vi "LVClient_up.vi"() -> ()   [LabVIEW 2018]
uses:
  <vilib>/picture/picture.llb/imagedata.ctl
panel:
  out "?":picture
  out "image data":T1
  in  "Stop Server":bool
  in  "Stop Client":bool
  in  "Init Button":bool
  in  "Play Button":bool
  out "Python server reply (9 bytes)":string
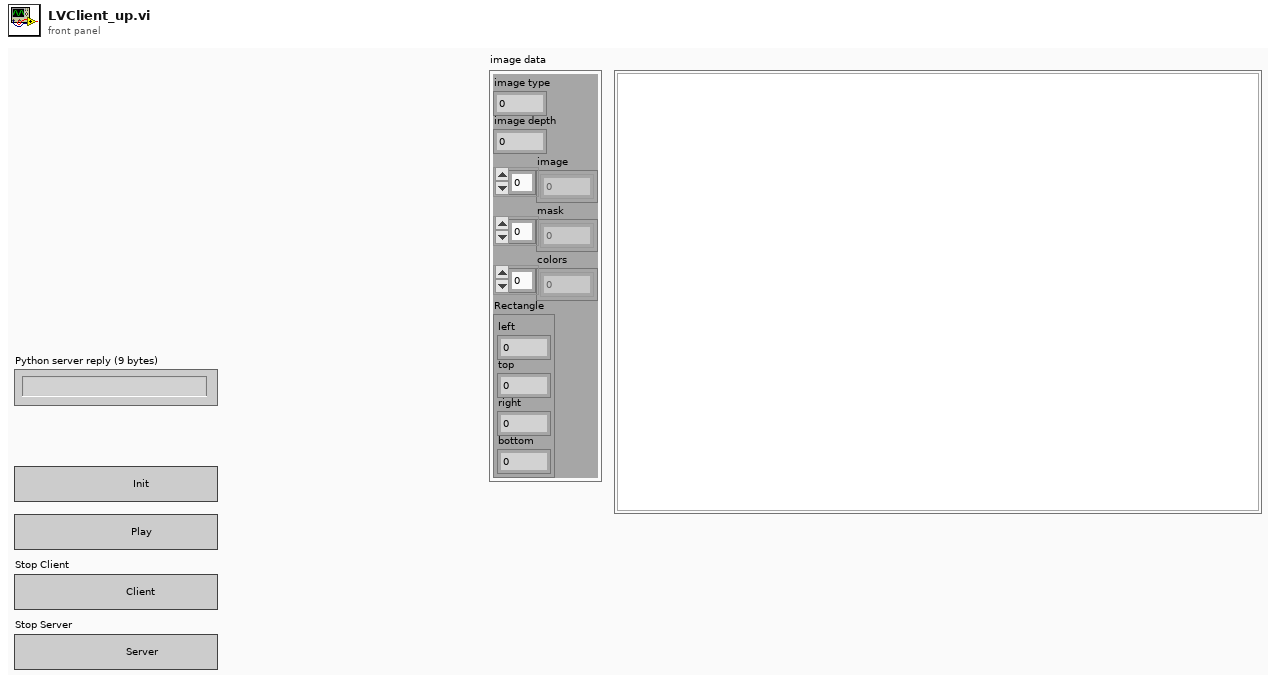
[diagram p1: front panel]
types:
  T1 = typedef "imagedata.ctl" = cluster{"image type":i32, "image depth":i32, "image":u8[], "mask":u8[], "colors":u32[], "Rectangle":cluster{"left":i16, "top":i16, "right":i16, "bottom":i16}}
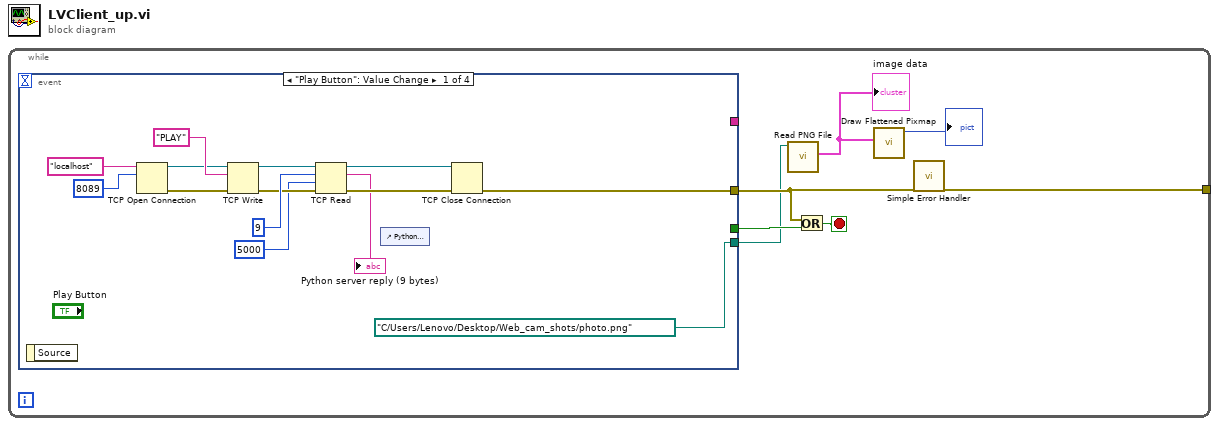
[diagram p0: block diagram]
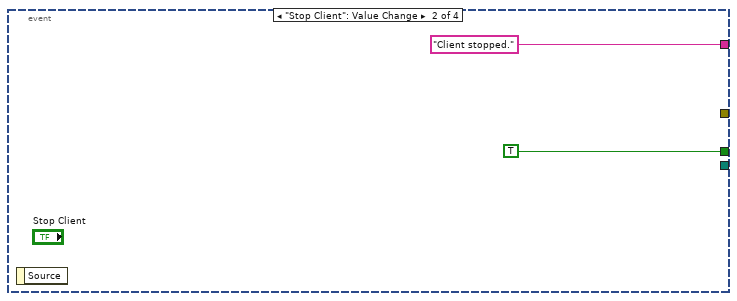
[diagram p2: hidden frame]
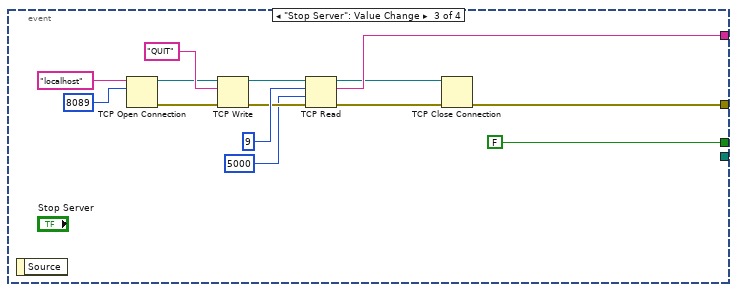
[diagram p3: hidden frame]
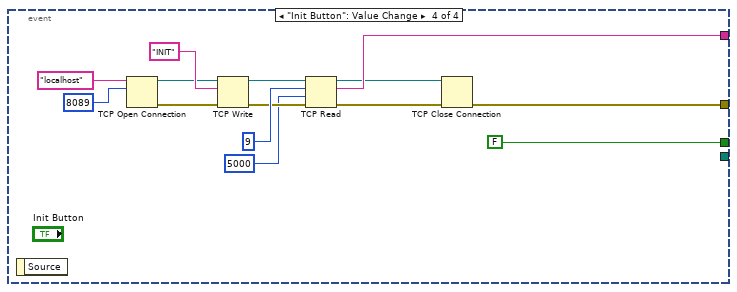
[diagram p4: hidden frame]
diagram:
  n1 = while {
    tunnel: [w7] -> w1
    stop <- w6 stop-if-true
    n2 = event shown="[0] \"Play Button\": Value Change" {
      selector: _ -> [_ _ _ _]
      dyn-events: _ -> [_ _ _ _]
      timeout: _ -> [_ _ _ _]
      tunnel: [w10 _ w25 w39] -> w7
      tunnel: [_ "Client stopped." ("data out") w32 w46] -> _
      tunnel: [_ TRUE FALSE FALSE] -> w5
      tunnel: [path "C:/Users/Lenovo/Desktop/Web_cam_shots/photo.png" _ _ _] -> w2
      event "Play Button": Value Change {
        n3 = event-data() -> ()  [unwired: 1 in, 1 out]
        n4 = TCP Open Connection(address="localhost", remote port or service name=u16 8089) -> (connection ID=w14:refnum<k5>, error out=w13:errorcluster)  [unwired: 3 in]
        n5 = TCP Write(connection ID=w14, data in="PLAY", error in (no error)=w13) -> (connection ID out=w19:refnum<k5>, error out=w18:errorcluster)  [unwired: 1 in, 1 out]
        n6 = TCP Read(connection ID=w19, bytes to read=9, error in (no error)=w18, 9:5000 ("timeout ms (25000)")) -> (connection ID out=w12:refnum<k5>, data out=→"Python server reply (9 bytes)":string, error out=w11:errorcluster)  [unwired: 1 in]
        n7 = control-ref of="Python server reply (9 bytes)"() -> ()  [unwired: 1 out]
        n8 = TCP Close Connection(connection ID=w12, error in (no error)=w11) -> (error out=w10:errorcluster)  [unwired: 1 in, 1 out]
      }
      event "Stop Client": Value Change {
        n9 = event-data() -> ()  [unwired: 1 in, 1 out]
      }
      event "Stop Server": Value Change {
        n10 = event-data() -> ()  [unwired: 1 in, 1 out]
        n11 = TCP Open Connection(address="localhost", remote port or service name=u16 8089) -> (connection ID=w29:refnum<k5>, error out=w28:errorcluster)  [unwired: 3 in]
        n12 = TCP Write(connection ID=w29, data in="QUIT", error in (no error)=w28) -> (connection ID out=w35:refnum<k5>, error out=w34:errorcluster)  [unwired: 1 in, 1 out]
        n13 = TCP Read(connection ID=w35, bytes to read=9, error in (no error)=w34, 9:5000 ("timeout ms (25000)")) -> (connection ID out=w27:refnum<k5>, data out=w32:string, error out=w26:errorcluster)  [unwired: 1 in]
        n14 = TCP Close Connection(connection ID=w27, error in (no error)=w26) -> (error out=w25:errorcluster)  [unwired: 1 in, 1 out]
      }
      event "Init Button": Value Change {
        n15 = event-data() -> ()  [unwired: 1 in, 1 out]
        n16 = TCP Open Connection(address="localhost", remote port or service name=u16 8089) -> (connection ID=w43:refnum<k5>, error out=w42:errorcluster)  [unwired: 3 in]
        n17 = TCP Write(connection ID=w43, data in="INIT", error in (no error)=w42) -> (connection ID out=w49:refnum<k5>, error out=w48:errorcluster)  [unwired: 1 in, 1 out]
        n18 = TCP Read(connection ID=w49, bytes to read=9, error in (no error)=w48, 9:5000 ("timeout ms (25000)")) -> (connection ID out=w41:refnum<k5>, data out=w46:string, error out=w40:errorcluster)  [unwired: 1 in]
        n19 = TCP Close Connection(connection ID=w41, error in (no error)=w40) -> (error out=w39:errorcluster)  [unwired: 1 in, 1 out]
      }
    }
    n20 = call <vilib>:"Read PNG File.vi"("path to PNG file"=w2) -> ("image data"=w4:T1)  [unwired: 8 in, 2 out]
    "image data" <- w4
    n21 = Or(x=w7, y=w5) -> (x .or. y?=w6:bool)
    n22 = call <vilib>:"Draw Flattened Pixmap.vi"("image data"=w4) -> ("new picture"=→"?":picture)  [unwired: 8 in]
  }
  n23 = call <vilib>:"Simple Error Handler.vi"("error in (no error)"=w1) -> ()  [unwired: 4 in, 5 out]
